vi "split_pixels.vi"(8 "error in (no error)":errorcluster, 10 "Channel index":i32, 11 "ImageAssemblerRK110612Spiral in":refnum<class "ImageAssemblerRK110612Spiral.lvclass">) -> (0 "error out":errorcluster, 1 "For next frame":dbl[](array[numeric]), 2 "Pixel block":sgl[](array[numeric]), 3 "ImageAssemblerRK110612Spiral out":refnum<class "ImageAssemblerRK110612Spiral.lvclass">, 4 "Next insertion position":i32, 5 "End of frame reached?":bool, 7 "Another frame possible?":bool)   [LabVIEW 2010, in "ImageAssemblerRK110612Spiral.lvclass"]
uses:
  ImageAssemblerRK110612Spiral.lvclass
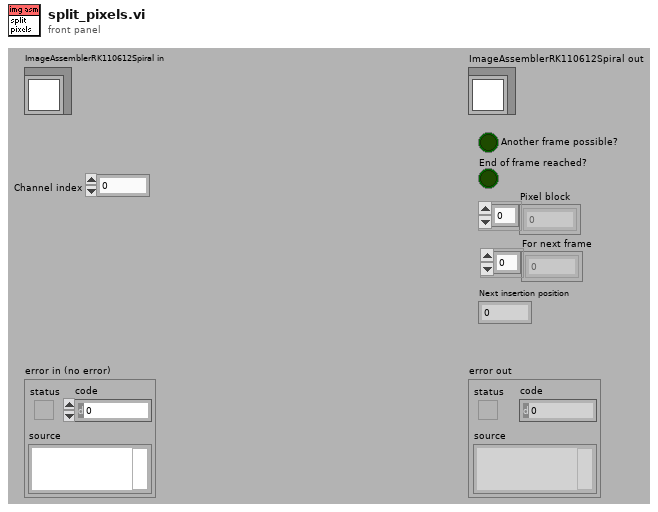
[diagram p1: front panel]
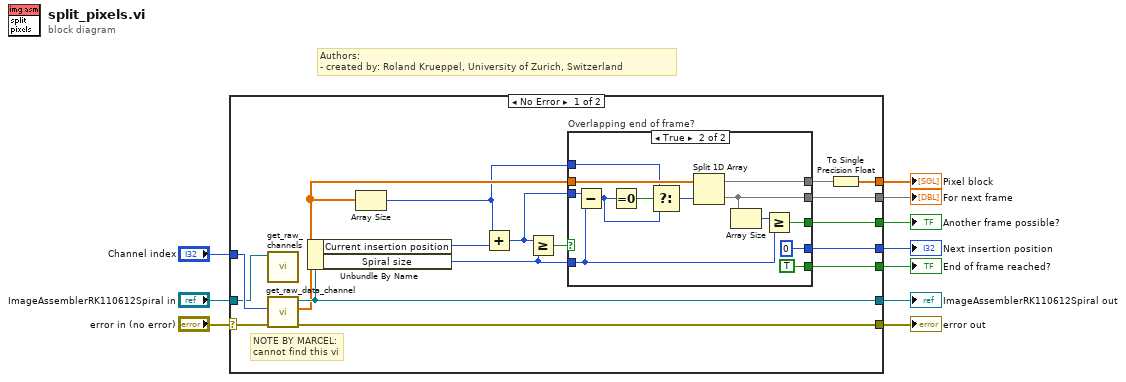
[diagram p0: block diagram]
diagram:
  # "Authors: \n- created by: Roland Krueppel, University of Zurich, Switzerland"
  n1 = case shown="No Error" "error in (no error)" {
    selector: "error in (no error)" -> [w27 w44]
    tunnel: [w26 w44] -> w9
    tunnel: [w25 w43] -> w7
    tunnel: "ImageAssemblerRK110612Spiral in" -> [w11 w43]
    tunnel: "Channel index" -> [w12 _]
    tunnel: [w23 _] -> w5
    tunnel: [w22 _] -> w4
    tunnel: [w15 _] -> w2
    tunnel: [w21 _] -> w3
    tunnel: [w13 _] -> w1
    frame No Error {
      # "NOTE BY MARCEL:\ncannot find this vi"
      n2 = call-dynamic "get_raw_channels.vi"("DL090211ImageAssemblerScaffold.lvclass in"=w11) -> ()  [unwired: 8 in, 3 out]
      n3 = call-dynamic "get_raw_data_channel.vi"("error in (no error)"=w27, "Channel index"=w12) -> ("error out"=w26:errorcluster, "raw data channel"=w17:dbl[], "GenericImageAssembler out"=w25:refnum<class "ImageAssemblerRK110612Spiral.lvclass">)  [unwired: 7 in]
      n4 = Unbundle By Name(w25) -> ("Current insertion position"=w18:i32, "Spiral size"=w20:i32)
      n5 = Array Size(array=w17) -> (size(s)=w14:i32)
      n6 = Add(x=w14, y=w18) -> (x+y=w19:i32)
      n7 = Greater Or Equal?(x=w19, y=w20) -> (x >= y?=w24:bool)
      n8 = case "Overlapping end of frame?" shown="True" w24 {
        tunnel: [_ TRUE] -> w23
        tunnel: [w29 0 ("Current insertion position")] -> w21
        tunnel: w20 -> [_ w31]
        tunnel: w19 -> [w29 w39]
        tunnel: w17 -> [w28 w40]
        tunnel: [w28 w38] -> w16
        tunnel: [_ w33] -> w15
        tunnel: w14 -> [_ w34]
        tunnel: [_ w30] -> w13
        frame False {
        }
        frame True {
          n9 = Subtract(x=w39, y=w31) -> (x-y=w36:i32)
          n10 = Equal To 0?(x=w36) -> (x = 0?=w37:bool)
          n11 = Select(t=w34, s=w37, f=w36) -> (s? t:f=w35:i32)
          n12 = Split 1D Array(array=w40, index=w35) -> (first subarray=w38:dbl[], second subarray=w33:dbl[])
          n13 = Array Size(array=w33) -> (size(s)=w32:i32)
          n14 = Greater Or Equal?(x=w32, y=w31) -> (x >= y?=w30:bool)
        }
      }
      n15 = To Single Precision Float(number=w16) -> (single precision float=w22:sgl[])
    }
    frame Error {
    }
  }
  "error out" <- w9
  "ImageAssemblerRK110612Spiral out" <- w7
  "End of frame reached?" <- w5
  "Pixel block" <- w4
  "For next frame" <- w2
  "Next insertion position" <- w3
  "Another frame possible?" <- w1
